vi "Read Data.vi"(0 "comm interface in":refnum<class "RoboRIO I2C.lvclass">, 5 "bytes to read":i32, 11 "error in":errorcluster) -> (4 "comm interface out":refnum<class "RoboRIO I2C.lvclass">, 6 "data":u8[](array[numeric]), 15 "error out":errorcluster)   [LabVIEW 2018, in "RoboRIO I2C.lvclass"]
uses:
  RoboRIO I2C.lvclass
  RoboRIO I2C.lvclass/RoboRIO I2C.ctl
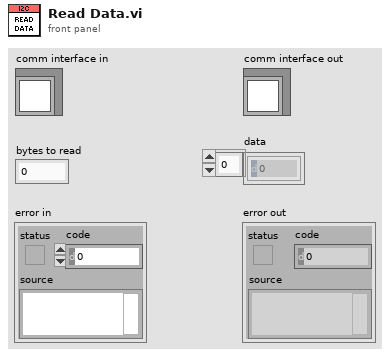
[diagram p1: front panel]
types:
  T1 = typedef "WPI_I2CDevRef.ctl" = cluster{"DevStatus":errorcluster, "Device Address":u8, "Handle":i32, "I2C Bus":T2}
  T2 = typedef "i2c_bus.ctl" = enum16{"I2C On-Board", "I2C MXP", "Invalid"}
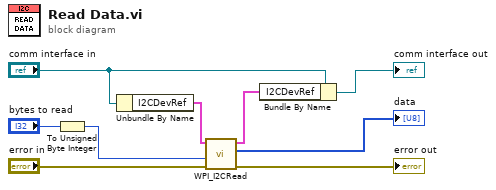
[diagram p0: block diagram]
diagram:
  n1 = To Unsigned Byte Integer(number="bytes to read") -> (unsigned 8bit integer=w4:u8)
  n2 = Unbundle By Name("comm interface in") -> ("I2CDevRef"=w6:T1)
  n3 = call <vilib>:"WPI_I2CRead.vi"("error in (no error)"="error in", "I2CBytesToRead"=w4, "I2CDevRef"=w6) -> ("error out"=→"error out":errorcluster, "Data Out"=→"data":u8[], "I2CDevRef"=w3:T1)  [unwired: 6 in]
  n4 = Bundle By Name(cluster="comm interface in", "I2CDevRef"=w3) -> (→"comm interface out":refnum<class "RoboRIO I2C.lvclass">)
